vi "PantherLAB_Log - Duplicate DQMH Module.vi"(4 "Original Tester":path, 6 "Original Library":path, 9 "New Tester":path, 10 "New Library":path, 11 "Project":refnum<vi>) -> (0 "error out":errorcluster)   [LabVIEW 2016]
doc: "_____\nCreated using DQMH Framework: Event Scripter 7.1.0.1450."
uses:
  PantherLAB Scripting Hooks/PantherLAB_Scripting.lvlib
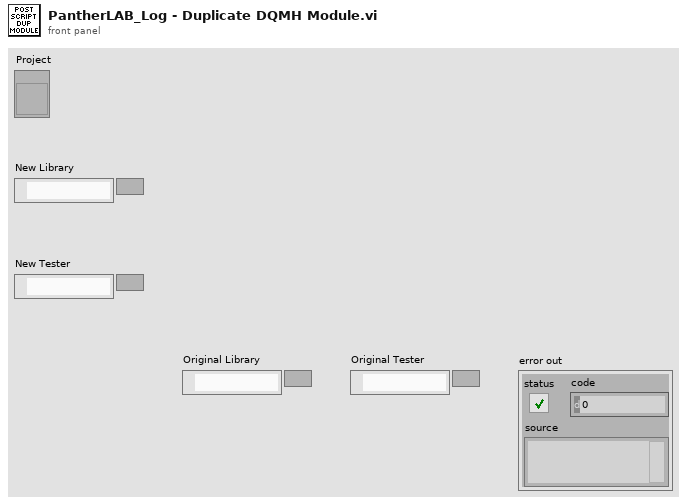
[diagram p1: front panel]
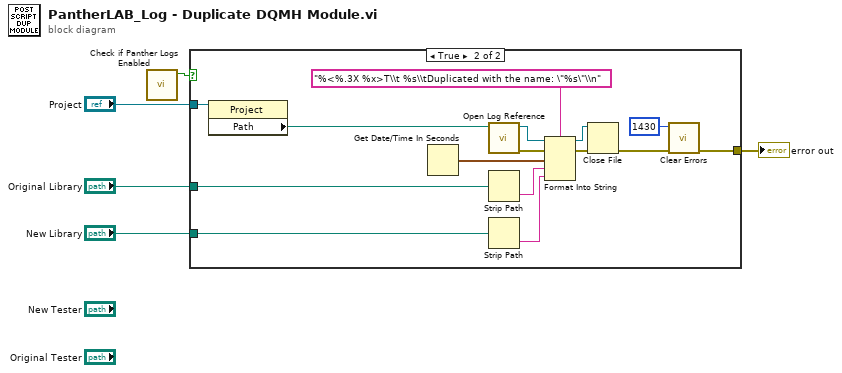
[diagram p0: block diagram]
diagram:
  n1 = call "Check if Panther Logs Enabled.vi"() -> ("PantherLogs Enabled?"=w4:bool)  [unwired: 11 in]
  n2 = case shown="True" w4 {
    tunnel: "Project" -> [_ w13]
    tunnel: "Original Library" -> [_ w11]
    tunnel: "New Library" -> [_ w8]
    tunnel: [_ w7] -> w5
    frame False {
    }
    frame True {
      n3 = property class="Project"(reference=w13) -> ("Path"=w14:path)  [unwired: 1 in, 2 out]
      n4 = Get Date/Time In Seconds() -> (seconds since 1Jan1904=w15:timestamp)
      n5 = call "Open Log Reference.vi"("Project Path"=w14) -> ("error out"=w20:errorcluster, "File Reference"=w17:refnum<file>)  [unwired: 9 in]
      n6 = Strip Path(path=w11) -> (name=w10:string)  [unwired: 1 out]
      n7 = Strip Path(path=w8) -> (name=w9:string)  [unwired: 1 out]
      n8 = Format Into String(format string="%<%.3X %x>T\\t %s\\tDuplicated with the name: \"%s\"\\n", initial string=w17, error in=w20, w15, w10, w9) -> (resulting string=w16:refnum<file>, error out=w19:errorcluster)
      n9 = Close File(refnum=w16, error in=w19) -> (error out=w18:errorcluster)  [unwired: 1 out]
      n10 = call <vilib>:"Clear Errors.vi"("error in (no error)"=w18, "specific error code to clear (0: all)"=1430) -> ("error out"=w7:errorcluster)  [unwired: 4 in, 1 out]
    }
  }
  "error out" <- w5
